vi "Part 1.vi"(11 "Input":string) -> (3 "Output":i64)   [LabVIEW 2021]
uses:
  <userlib>/_OpenG.lib/string/string.llb/Convert EOLs (String)__ogtk.vi
panel:
  out "Polygon":cluster{i32, i32}[](array[cluster])
  out "Array":string[][](array[string])
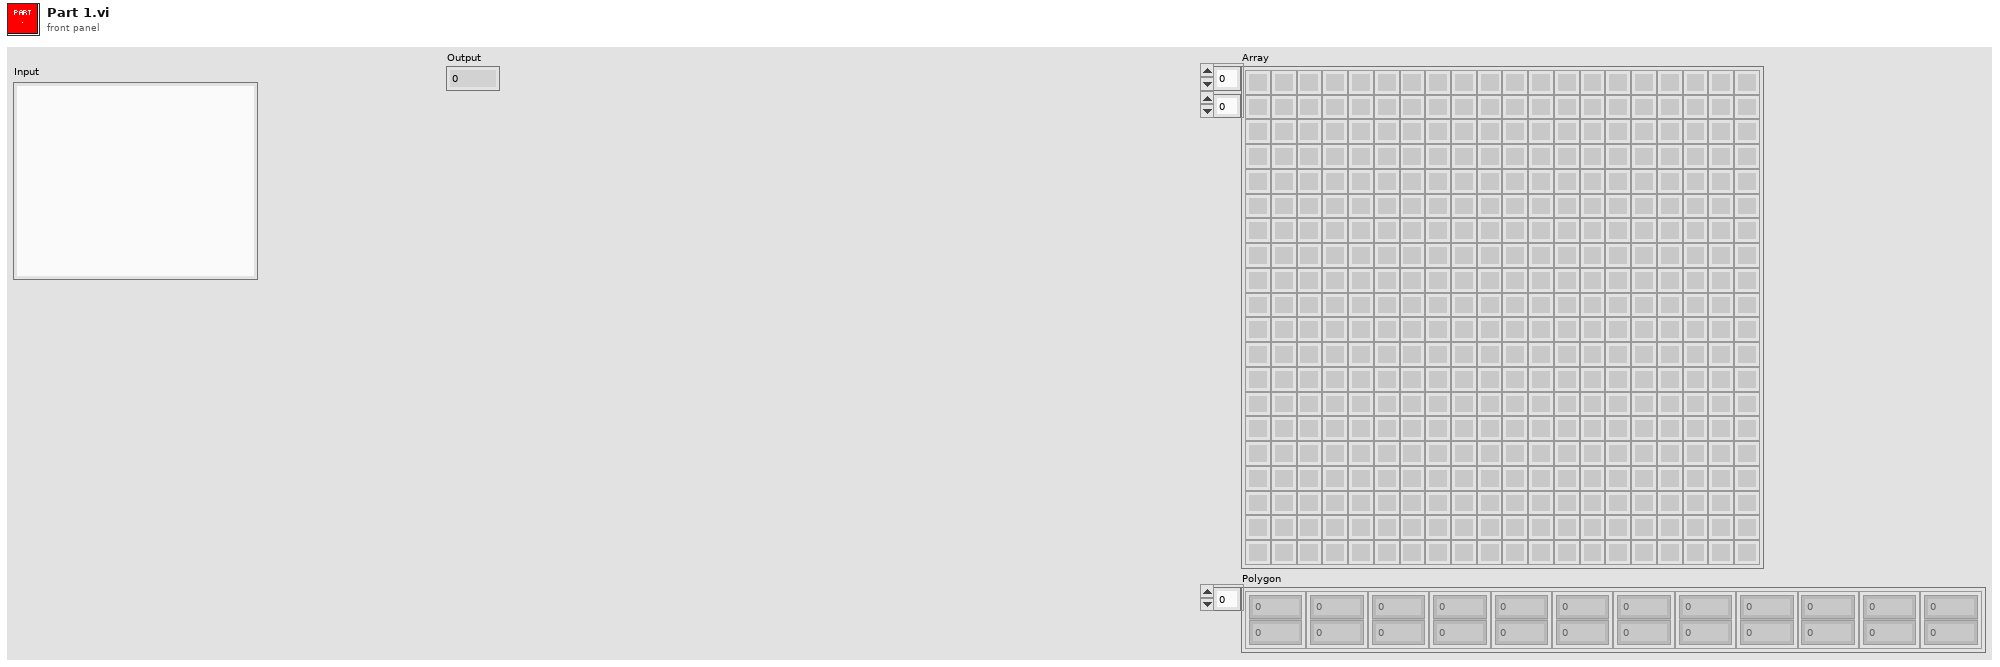
[diagram p1: front panel]
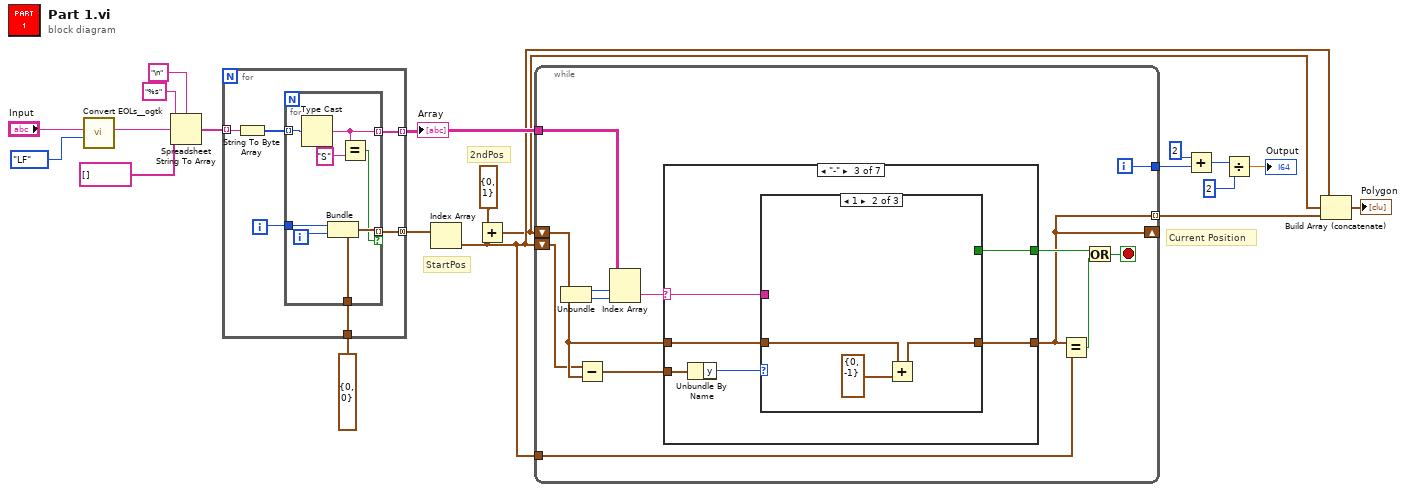
[diagram p0: block diagram]
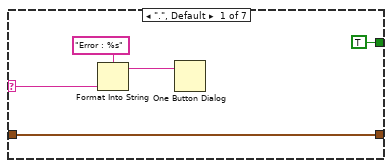
[diagram p2: hidden frame]
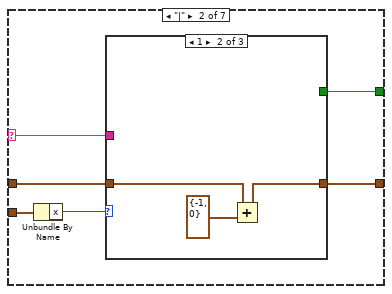
[diagram p3: hidden frame]
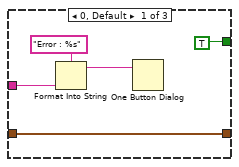
[diagram p4: hidden frame]
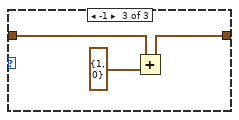
[diagram p5: hidden frame]
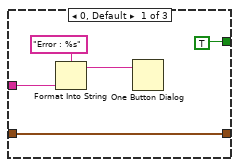
[diagram p6: hidden frame]
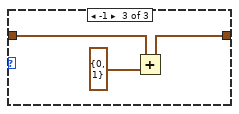
[diagram p7: hidden frame]
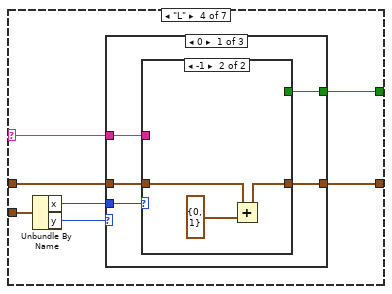
[diagram p8: hidden frame]
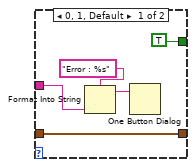
[diagram p9: hidden frame]
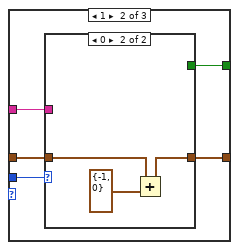
[diagram p10: hidden frame]
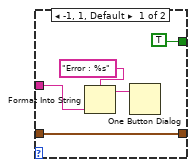
[diagram p11: hidden frame]
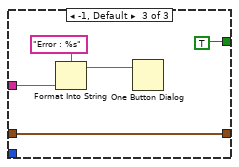
[diagram p12: hidden frame]
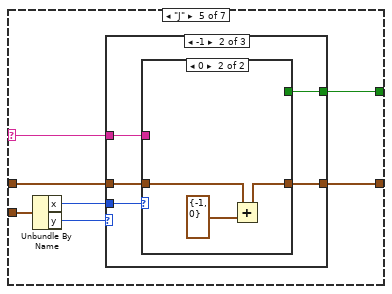
[diagram p13: hidden frame]
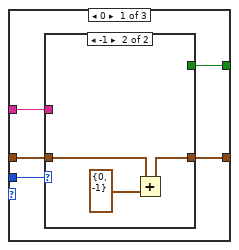
[diagram p14: hidden frame]
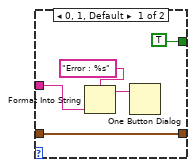
[diagram p15: hidden frame]
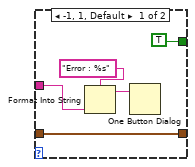
[diagram p16: hidden frame]
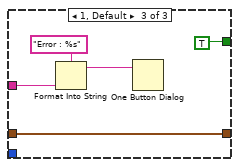
[diagram p17: hidden frame]
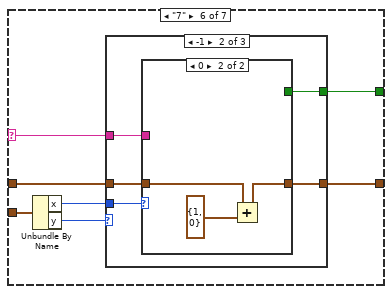
[diagram p18: hidden frame]
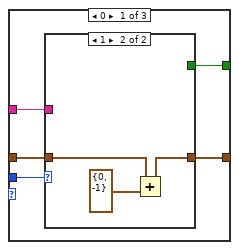
[diagram p19: hidden frame]
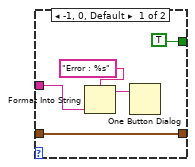
[diagram p20: hidden frame]
diagram:
  # "2ndPos"
  # "StartPos"
  # "Current Position"
  n1 = call-poly <userlib>:"Convert EOLs__ogtk.vi"("Convert to:"=enum16{"CR", "LF", "CRLF"}."LF", "String in"="Input") -> ("String out"=w16:string)  [unwired: 9 in]
  n2 = Spreadsheet String To Array(delimiter (Tab)="\n", format string="%s", spreadsheet string=w16, array type (2D Dbl)=string[] []) -> (array=w14:string[])
  n3 = for {
    tunnel: w14 -> [w26] mode=indexing
    tunnel: [w24] -> w8 mode=indexing
    tunnel: [w22] -> w13 mode=concatenating
    tunnel: cluster{"x":i32, "y":i32} {"x"=0, "y"=0} ("cluster") -> [w21]
    i -> [w23]
    n4 = String To Byte Array(string=w26) -> (unsigned byte array=w25:u8[])
    n5 = for {
      tunnel: w25 -> [w34] mode=indexing
      tunnel: [w33] -> w24 mode=indexing
      tunnel: w23 -> [w30]
      tunnel: [w29] -> w22 mode=indexing if=w28
      tunnel: w21 -> [w27]
      i -> [w31]
      n6 = Type Cast(x=w34) -> (*(type *) &x=w33:string)  [unwired: 1 in]
      n7 = Bundle(cluster=w27, "x"=w30, "y"=w31) -> (w29:cluster{"x":i32, "y":i32})
      n8 = Equal?(x=w33, y="S") -> (x = y?=w28:bool)
    }
  }
  "Array" <- w8
  n9 = Index Array(array=w13) -> (element=w4:cluster{"x":i32, "y":i32})  [unwired: 1 in]
  n10 = Add(x=cluster{i32, i32} {0, 1} ("y"), y=w4) -> (x+y=w3:cluster{i32, i32})
  n11 = while {
    shift-right: [w35] -> _
    shift-left: w3 -> [w41]
    shift-left: w4 -> [w40]
    tunnel: w4 -> [w47]
    tunnel: [w46] -> w12
    tunnel: w8 -> [w45]
    tunnel: [w35] -> w5 mode=indexing
    i -> [w46]
    stop <- w38 stop-if-true
    n12 = Unbundle(w41) -> ("x"=w44:i32, "y"=w43:i32)
    n13 = Subtract(x=w40, y=w41) -> (x-y=w39:cluster{"x":i32, "y":i32})
    n14 = Index Array(array=w45, index (row)=w44, index (col)=w43) -> (element=w42:string)
    n15 = case shown="\"-\"" w42 {
      selector: w42 -> [w50 w53 w71 w89 w127 w165 w203]
      tunnel: w41 -> [w52 w56 w74 w92 w130 w168 w206]
      tunnel: [w52 w55 w73 w91 w129 w167 w205] -> w35
      tunnel: w39 -> [_ w58 w75 w93 w131 w169 w207]
      tunnel: [TRUE w54 w72 w90 w128 w166 w204] -> w37
      frame ".", Default {
        n16 = Format Into String(format string="Error : %s" ("message"), w50) -> (resulting string=w49:string)  [unwired: 2 in, 1 out]
        n17 = One Button Dialog(message=w49) -> ()  [unwired: 1 in, 1 out]
      }
      frame "|" {
        n18 = Unbundle By Name(w58) -> ("x"=w57:i32)
        n19 = case shown="1" w57 {
          tunnel: w56 -> [w63 w66 w69]
          tunnel: [w63 w65 w68] -> w55
          tunnel: [TRUE _ _] -> w54
          tunnel: w53 -> [w60 _ _]
          frame 0, Default {
            n20 = Format Into String(format string="Error : %s" ("message"), w60) -> (resulting string=w61:string)  [unwired: 2 in, 1 out]
            n21 = One Button Dialog(message=w61) -> ()  [unwired: 1 in, 1 out]
          }
          frame 1 {
            n22 = Add(x=w66, y=cluster{i32, i32} {-1, 0}) -> (x+y=w65:cluster{i32, i32})
          }
          frame -1 {
            n23 = Add(x=w69, y=cluster{i32, i32} {1, 0}) -> (x+y=w68:cluster{i32, i32})
          }
        }
      }
      frame "-" {
        n24 = Unbundle By Name(w75) -> ("y"=w70:i32)
        n25 = case shown="1" w70 {
          tunnel: w74 -> [w80 w83 w86]
          tunnel: [w80 w82 w85] -> w73
          tunnel: [TRUE _ _] -> w72
          tunnel: w71 -> [w77 _ _]
          frame 0, Default {
            n26 = Format Into String(format string="Error : %s" ("message"), w77) -> (resulting string=w78:string)  [unwired: 2 in, 1 out]
            n27 = One Button Dialog(message=w78) -> ()  [unwired: 1 in, 1 out]
          }
          frame 1 {
            n28 = Add(x=w83, y=cluster{i32, i32} {0, -1}) -> (x+y=w82:cluster{i32, i32})
          }
          frame -1 {
            n29 = Add(x=w86, y=cluster{i32, i32} {0, 1}) -> (x+y=w85:cluster{i32, i32})
          }
        }
      }
      frame "L" {
        n30 = Unbundle By Name(w93) -> ("x"=w87:i32, "y"=w88:i32)
        n31 = case shown="0" w88 {
          tunnel: w92 -> [w98 w111 w124]
          tunnel: [w97 w110 w124] -> w91
          tunnel: [w95 w108 TRUE] -> w90
          tunnel: w89 -> [w94 w107 w121]
          tunnel: w87 -> [w96 w109 _]
          frame 0 {
            n32 = case shown="-1" w96 {
              tunnel: w98 -> [w103 w106]
              tunnel: [w103 w105] -> w97
              tunnel: [TRUE _] -> w95
              tunnel: w94 -> [w99 _]
              frame 0, 1, Default {
                n33 = Format Into String(format string="Error : %s" ("message"), w99) -> (resulting string=w101:string)  [unwired: 2 in, 1 out]
                n34 = One Button Dialog(message=w101) -> ()  [unwired: 1 in, 1 out]
              }
              frame -1 {
                n35 = Add(x=w106, y=cluster{i32, i32} {0, 1}) -> (x+y=w105:cluster{i32, i32})
              }
            }
          }
          frame 1 {
            n36 = case shown="0" w109 {
              tunnel: w111 -> [w116 w119]
              tunnel: [w116 w118] -> w110
              tunnel: [TRUE _] -> w108
              tunnel: w107 -> [w112 _]
              frame -1, 1, Default {
                n37 = Format Into String(format string="Error : %s" ("message"), w112) -> (resulting string=w114:string)  [unwired: 2 in, 1 out]
                n38 = One Button Dialog(message=w114) -> ()  [unwired: 1 in, 1 out]
              }
              frame 0 {
                n39 = Add(x=w119, y=cluster{i32, i32} {-1, 0}) -> (x+y=w118:cluster{i32, i32})
              }
            }
          }
          frame -1, Default {
            n40 = Format Into String(format string="Error : %s" ("message"), w121) -> (resulting string=w122:string)  [unwired: 2 in, 1 out]
            n41 = One Button Dialog(message=w122) -> ()  [unwired: 1 in, 1 out]
          }
        }
      }
      frame "J" {
        n42 = Unbundle By Name(w131) -> ("x"=w125:i32, "y"=w126:i32)
        n43 = case shown="-1" w126 {
          tunnel: w130 -> [w136 w149 w162]
          tunnel: [w135 w148 w162] -> w129
          tunnel: [w133 w146 TRUE] -> w128
          tunnel: w127 -> [w132 w145 w159]
          tunnel: w125 -> [w134 w147 _]
          frame 0 {
            n44 = case shown="-1" w134 {
              tunnel: w136 -> [w141 w144]
              tunnel: [w141 w143] -> w135
              tunnel: [TRUE _] -> w133
              tunnel: w132 -> [w137 _]
              frame 0, 1, Default {
                n45 = Format Into String(format string="Error : %s" ("message"), w137) -> (resulting string=w139:string)  [unwired: 2 in, 1 out]
                n46 = One Button Dialog(message=w139) -> ()  [unwired: 1 in, 1 out]
              }
              frame -1 {
                n47 = Add(x=w144, y=cluster{i32, i32} {0, -1}) -> (x+y=w143:cluster{i32, i32})
              }
            }
          }
          frame -1 {
            n48 = case shown="0" w147 {
              tunnel: w149 -> [w154 w157]
              tunnel: [w154 w156] -> w148
              tunnel: [TRUE _] -> w146
              tunnel: w145 -> [w150 _]
              frame -1, 1, Default {
                n49 = Format Into String(format string="Error : %s" ("message"), w150) -> (resulting string=w152:string)  [unwired: 2 in, 1 out]
                n50 = One Button Dialog(message=w152) -> ()  [unwired: 1 in, 1 out]
              }
              frame 0 {
                n51 = Add(x=w157, y=cluster{i32, i32} {-1, 0}) -> (x+y=w156:cluster{i32, i32})
              }
            }
          }
          frame 1, Default {
            n52 = Format Into String(format string="Error : %s" ("message"), w159) -> (resulting string=w160:string)  [unwired: 2 in, 1 out]
            n53 = One Button Dialog(message=w160) -> ()  [unwired: 1 in, 1 out]
          }
        }
      }
      frame "7" {
        n54 = Unbundle By Name(w169) -> ("x"=w163:i32, "y"=w164:i32)
        n55 = case shown="-1" w164 {
          tunnel: w168 -> [w174 w187 w200]
          tunnel: [w173 w186 w200] -> w167
          tunnel: [w171 w184 TRUE] -> w166
          tunnel: w165 -> [w170 w183 w197]
          tunnel: w163 -> [w172 w185 _]
          frame 0 {
            n56 = case shown="1" w172 {
              tunnel: w174 -> [w179 w182]
              tunnel: [w179 w181] -> w173
              tunnel: [TRUE _] -> w171
              tunnel: w170 -> [w175 _]
              frame -1, 0, Default {
                n57 = Format Into String(format string="Error : %s" ("message"), w175) -> (resulting string=w177:string)  [unwired: 2 in, 1 out]
                n58 = One Button Dialog(message=w177) -> ()  [unwired: 1 in, 1 out]
              }
              frame 1 {
                n59 = Add(x=w182, y=cluster{i32, i32} {0, -1}) -> (x+y=w181:cluster{i32, i32})
              }
            }
          }
          frame -1 {
            n60 = case shown="0" w185 {
              tunnel: w187 -> [w192 w195]
              tunnel: [w192 w194] -> w186
              tunnel: [TRUE _] -> w184
              tunnel: w183 -> [w188 _]
              frame -1, 1, Default {
                n61 = Format Into String(format string="Error : %s" ("message"), w188) -> (resulting string=w190:string)  [unwired: 2 in, 1 out]
                n62 = One Button Dialog(message=w190) -> ()  [unwired: 1 in, 1 out]
              }
              frame 0 {
                n63 = Add(x=w195, y=cluster{i32, i32} {1, 0}) -> (x+y=w194:cluster{i32, i32})
              }
            }
          }
          frame 1, Default {
            n64 = Format Into String(format string="Error : %s" ("message"), w197) -> (resulting string=w198:string)  [unwired: 2 in, 1 out]
            n65 = One Button Dialog(message=w198) -> ()  [unwired: 1 in, 1 out]
          }
        }
      }
      frame "F" {
        n66 = Unbundle By Name(w207) -> ("x"=w201:i32, "y"=w202:i32)
        n67 = case shown="1" w202 {
          tunnel: w206 -> [w212 w225 w238]
          tunnel: [w211 w224 w238] -> w205
          tunnel: [w209 w222 TRUE] -> w204
          tunnel: w203 -> [w208 w221 w235]
          tunnel: w201 -> [w210 w223 _]
          frame 0 {
            n68 = case shown="1" w210 {
              tunnel: w212 -> [w217 w220]
              tunnel: [w217 w219] -> w211
              tunnel: [TRUE _] -> w209
              tunnel: w208 -> [w213 _]
              frame -1, 0, Default {
                n69 = Format Into String(format string="Error : %s" ("message"), w213) -> (resulting string=w215:string)  [unwired: 2 in, 1 out]
                n70 = One Button Dialog(message=w215) -> ()  [unwired: 1 in, 1 out]
              }
              frame 1 {
                n71 = Add(x=w220, y=cluster{i32, i32} {0, 1}) -> (x+y=w219:cluster{i32, i32})
              }
            }
          }
          frame 1 {
            n72 = case shown="0" w223 {
              tunnel: w225 -> [w230 w233]
              tunnel: [w230 w232] -> w224
              tunnel: [TRUE _] -> w222
              tunnel: w221 -> [w226 _]
              frame -1, 1, Default {
                n73 = Format Into String(format string="Error : %s" ("message"), w226) -> (resulting string=w228:string)  [unwired: 2 in, 1 out]
                n74 = One Button Dialog(message=w228) -> ()  [unwired: 1 in, 1 out]
              }
              frame 0 {
                n75 = Add(x=w233, y=cluster{i32, i32} {1, 0}) -> (x+y=w232:cluster{i32, i32})
              }
            }
          }
          frame -1, Default {
            n76 = Format Into String(format string="Error : %s" ("message"), w235) -> (resulting string=w236:string)  [unwired: 2 in, 1 out]
            n77 = One Button Dialog(message=w236) -> ()  [unwired: 1 in, 1 out]
          }
        }
      }
    }
    n78 = Equal?(x=w35, y=w47) -> (x = y?=w36:bool)
    n79 = Or(x=w37, y=w36) -> (x .or. y?=w38:bool)
  }
  n80 = Add(x=2, y=w12) -> (x+y=w10:i32)
  n81 = Divide(x=w10, y=2) -> (x/y=→"Output":dbl)
  n82 = Build Array (concatenate)(w4, w3, w5) -> (→"Polygon":cluster{"x":i32, "y":i32}[])
